vi "Ethernet Open.vi"(8 "error in (no error)":errorcluster {"code" format="%.0x"}, 10 "Ethernet Config":T1={"IP Address"=[192, 168, 0, 1], "Port No"=24691}, 11 "Device ID (0)":i32) -> (0 "error out":errorcluster {"code" format="%.0x"}, 2 "Return Code":i32, 3 "Device ID out":i32)   [LabVIEW 2020, in "KEYENCE LJ-X8000A.lvlib"]
uses:
  KEYENCE LJ-X8000A.lvlib
  Clusters/Ethernet Config.ctl
panel:
  # "(c) 2019 KEYENCE CORPORATION.  ALL RIGHTS RESERVED."
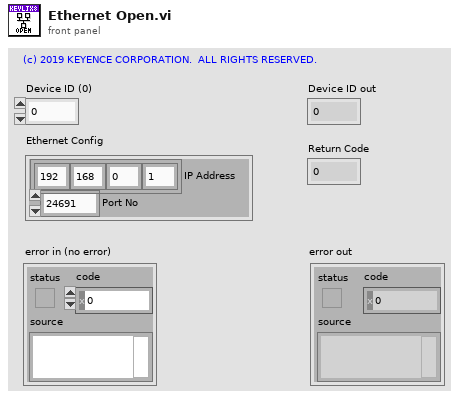
[diagram p1: front panel]
types:
  T1 = typedef "KEYENCE LJ-X8000A.lvlib/Ethernet Config.ctl" = cluster{"IP Address":u8[], "Port No":u16}
  T2 = cluster{"IP Address[0]":u8, "IP Address[1]":u8, "IP Address[2]":u8, "IP Address[3]":u8}
  T3 = cluster{"IP Address":cluster{"IP Address[0]":u8, "IP Address[1]":u8, "IP Address[2]":u8, "IP Address[3]":u8}, "Port No":u16, "reserved":u8, "reserved":u8}
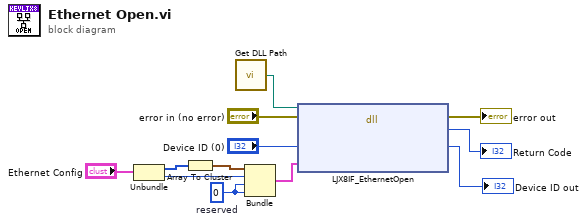
[diagram p0: block diagram]
diagram:
  w3 = u8 0  # reserved
  n1 = Unbundle("Ethernet Config") -> ("IP Address"=w6:u8[], "Port No"=w4:u16)
  n2 = Array To Cluster(array=w6) -> (cluster=w5:T2)
  n3 = call "Get DLL Path.vi"() -> ("DLL Path"=w1:path)  [unwired: 3 in]
  n4 = Bundle("IP Address"=w5, "Port No"=w4, "reserved"=w3, "reserved"=w3) -> (w2:T3)  [unwired: 1 in]
  n5 = dll-call lib="C:/Program Files (x86)/National Instruments/LabVIEW 2018/instr.lib/KEYENCE LJ-X8000/LJX8_IF.*" fn="LJX8IF_EthernetOpen"(path in=w1, error in="error in (no error)", "lDeviceId"="Device ID (0)", "pEthernetConfig"=w2) -> (error out=→"error out":errorcluster, "lRetCode"=→"Return Code":i32, "lDeviceId"=→"Device ID out":i32)  [unwired: 2 in, 1 out]
